vi "Write configuration.vi"(8 "error in":errorcluster, 10 "configuration":refnum<class "NISE_CEF_serializable configuration.lvclass">, 11 "System Diagnostics editor node in":refnum<class "System Diagnostics editor node.lvclass">) -> (0 "error out":errorcluster, 3 "System Diagnostics editor node out":refnum<class "System Diagnostics editor node.lvclass">)   [LabVIEW 2013, in "System Diagnostics editor node.lvclass"]
uses:
  System Diagnostics editor node.lvclass
  <vilib>/NI/Configuration Framework/serializable configuration/NISE_CEF_serializable configuration.lvclass
  module/configuration/System Diagnostics configuration.lvclass
  System Diagnostics editor node.lvclass/System Diagnostics editor node.ctl
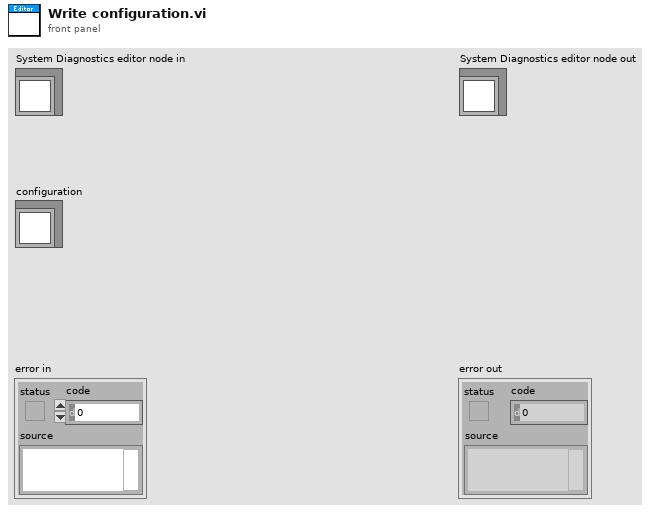
[diagram p1: front panel]
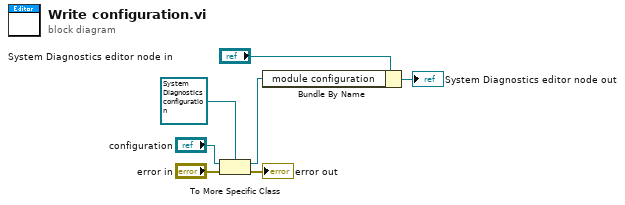
[diagram p0: block diagram]
diagram:
  n1 = To More Specific Class(target class=refnum<class "System Diagnostics configuration.lvclass"> refnum ("module configuration"), reference="configuration", error in="error in") -> (specific class reference=w1:refnum<class "System Diagnostics configuration.lvclass">, error out=→"error out":errorcluster)
  n2 = Bundle By Name(cluster="System Diagnostics editor node in", "module configuration"=w1) -> (→"System Diagnostics editor node out":refnum<class "System Diagnostics editor node.lvclass">)
